vi "Handle Mouse Down.vi"(4 "PlatMods":T2, 6 "Mods":cluster{"Double Click":bool, "Menu Key":bool}, 8 "error in (no error)":errorcluster, 9 "Button":u16, 10 "Coords":T3, 11 "Process Builder View in":refnum<class "Process Builder View.lvclass">) -> (0 "error out":errorcluster, 2 "Mouse Down Filtered Event Data":T1, 3 "Process Builder View out":refnum<class "Process Builder View.lvclass">)   [LabVIEW 2019, in "Process Builder View.lvclass"]
uses:
  <vilib>/gpm_packages/@cs/Car-wash/Source/Process Builder View/Process Builder View.lvclass
  C:/Program Files/National Instruments/LabVIEW 2019/vi.lib/gpm_packages/@cs/Test-executive-builder/Source/Test Executive Builder View/Test Executive Builder View/Test Executive Builder View.lvclass
  <vilib>/Utility/miscctls.llb/LVPoint32TypeDef.ctl
  <vilib>/gpm_packages/@cs/Test-executive-builder/Source/Application Dependencies/Mouse Down Filtered Event Data.ctl
  <vilib>/gpm_packages/@cs/Test-executive-builder/Source/Test Executive Builder View/Test Executive Builder View/Test Executive Builder View.lvclass/Test Executive Builder View.ctl
  <vilib>/gpm_packages/@cs/Test-executive-builder/Source/Test Executive Builder View/Test Executive Builder View/Test Executive Builder View.lvclass
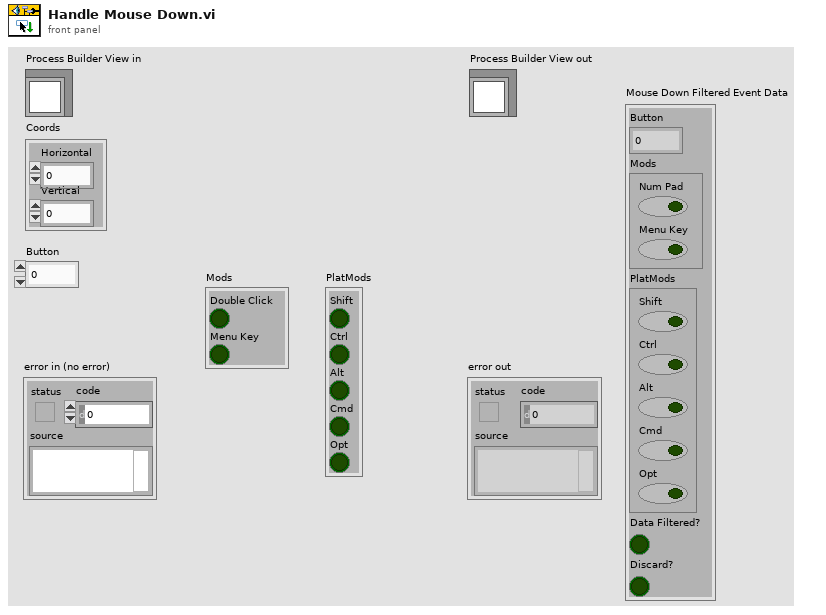
[diagram p1: front panel]
types:
  T1 = typedef "Mouse Down Filtered Event Data.ctl" = cluster{"Button":u16, "Mods":cluster{"Num Pad":bool, "Menu Key":bool}, "PlatMods":cluster{"Shift":bool, "Ctrl":bool, "Alt":bool, "Cmd":bool, "Opt":bool}, "Data Filtered?":bool, "Discard?":bool}
  T2 = cluster{"Shift":bool, "Ctrl":bool, "Alt":bool, "Cmd":bool, "Opt":bool}
  T3 = typedef "LVPoint32TypeDef.ctl" = cluster{"Horizontal":i32, "Vertical":i32}
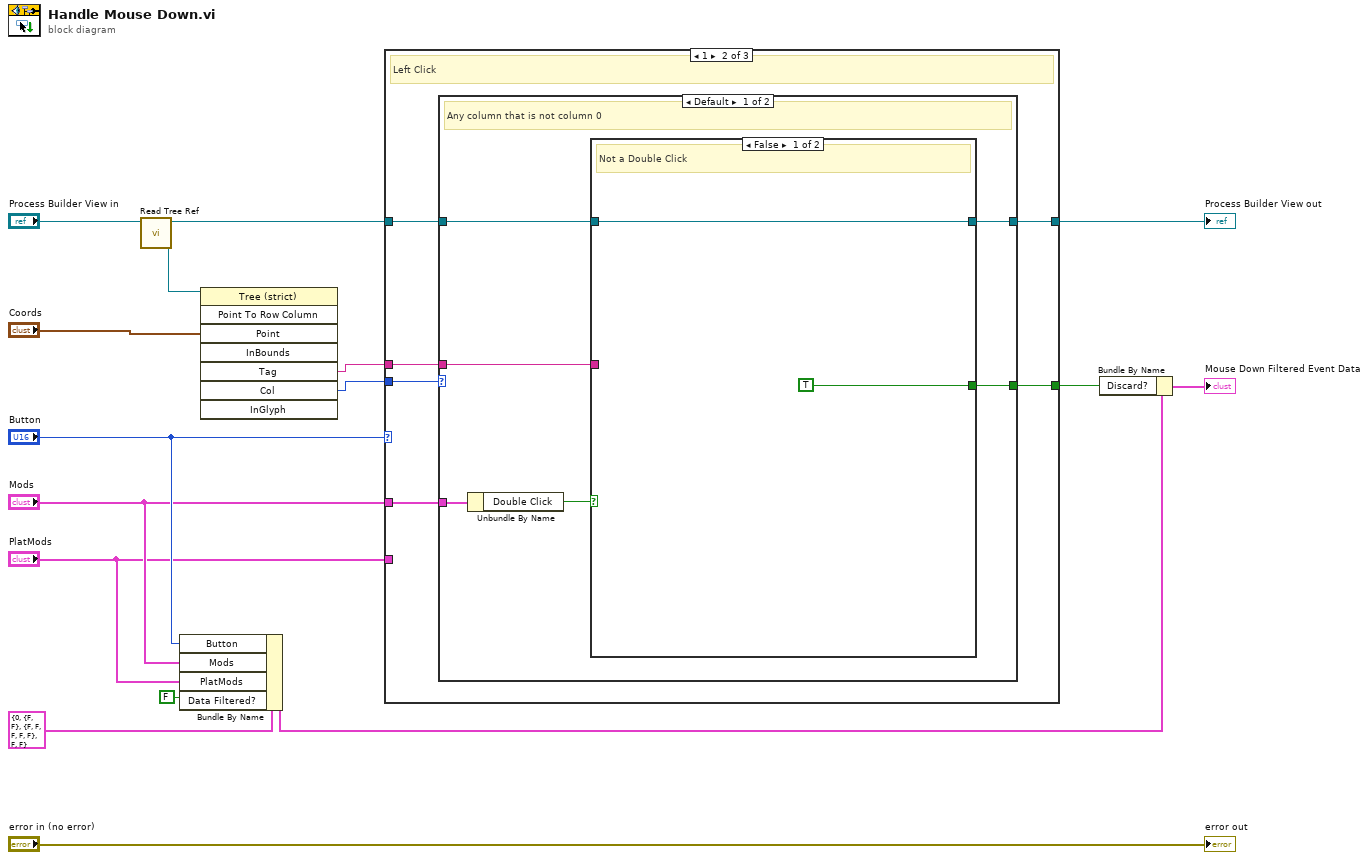
[diagram p0: block diagram]
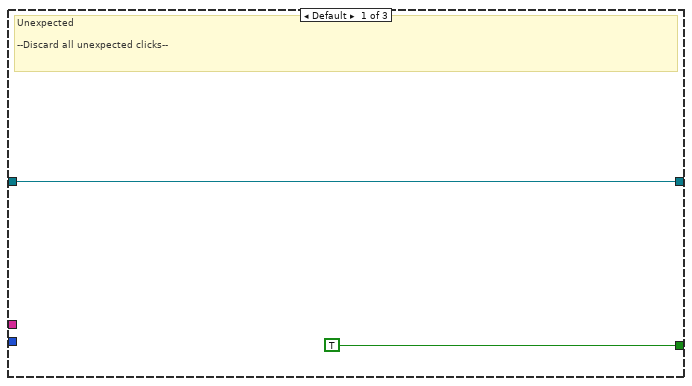
[diagram p2: hidden frame]
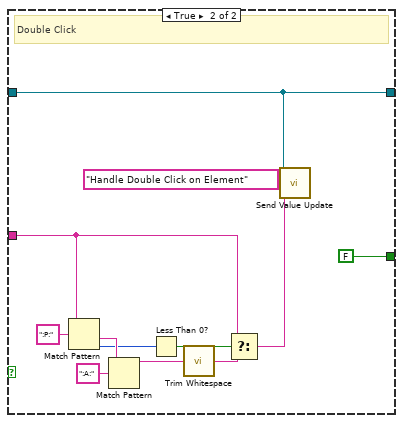
[diagram p3: hidden frame]
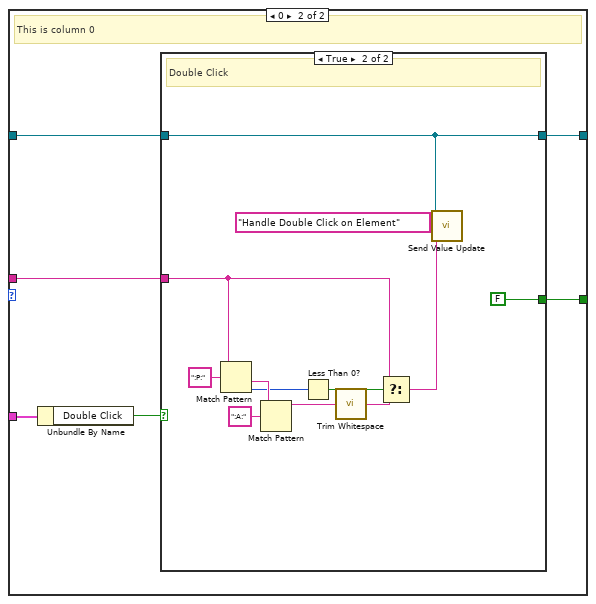
[diagram p4: hidden frame]
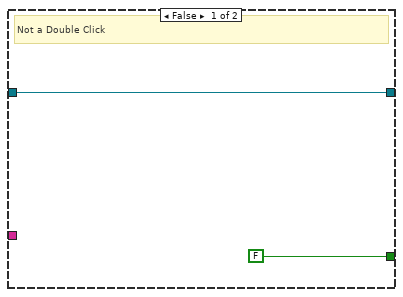
[diagram p5: hidden frame]
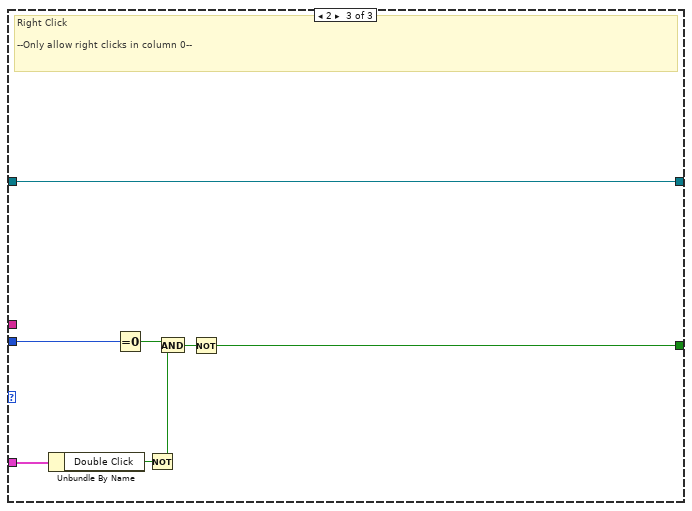
[diagram p6: hidden frame]
diagram:
  n1 = call <vilib>:"Read Tree Ref.vi"("Test Executive Builder View in"="Process Builder View in") -> ("Tree Ref"=w16:refnum<vi>, "Test Executive Builder View out"=w9:refnum<class "Process Builder View.lvclass">)  [unwired: 9 in]
  n2 = Bundle By Name(cluster=T1 {"Button"=0, "Mods"={"Num Pad"=FALSE, "Menu Key"=FALSE}, "PlatMods"={"Shift"=FALSE, "Ctrl"=FALSE, "Alt"=FALSE, "Cmd"=FALSE, "Opt"=FALSE}, "Data Filtered?"=FALSE, "Discard?"=FALSE} ("Mouse Down Filtered Event Data"), "Button"="Button", "Mods"="Mods", "PlatMods"="PlatMods", "Data Filtered?"=FALSE) -> (w12:T1)
  n3 = invoke class="Tree (strict)" method="Point To Row Column"(reference=w16, "Point"="Coords") -> ("Tag"=w14:string, "Col"=w15:i32)  [unwired: 6 in, 6 out]
  n4 = case shown="1" "Button" {
    tunnel: w15 -> [_ w24 w72]
    tunnel: w14 -> [_ w19 _]
    tunnel: "Mods" -> [_ w23 w70]
    tunnel: "PlatMods" -> [_ _ _]
    tunnel: [TRUE w22 w66] -> w10
    tunnel: w9 -> [w17 w21 w65]
    tunnel: [w17 w20 w65] -> w7
    frame Default {
      # "Unexpected\n\n--Discard all unexpected clicks--"
    }
    frame 1 {
      # "Left Click"
      n5 = case shown="Default" w24 {
        tunnel: w23 -> [w30 w50]
        tunnel: [w28 w48] -> w22
        tunnel: w21 -> [w26 w46]
        tunnel: [w27 w47] -> w20
        tunnel: w19 -> [w25 w45]
        frame Default {
          # "Any column that is not column 0"
          n6 = Unbundle By Name(w30) -> ("Double Click"=w29:bool)
          n7 = case shown="False" w29 {
            tunnel: [TRUE FALSE] -> w28
            tunnel: [w31 w35] -> w27
            tunnel: w26 -> [w31 w35]
            tunnel: w25 -> [_ w36]
            frame False {
              # "Not a Double Click"
            }
            frame True {
              # "Double Click"
              n8 = Match Pattern(string=w36, regular expression=":P:") -> (after substring=w42:string, offset past match=w41:i32)  [unwired: 1 in, 2 out]
              n9 = Match Pattern(string=w42, regular expression=":A:") -> (before substring=w40:string)  [unwired: 1 in, 3 out]
              n10 = Less Than 0?(x=w41) -> (x < 0?=w38:bool)
              n11 = call <vilib>:"Trim Whitespace.vi"("string"=w40) -> ("trimmed string"=w37:string)  [unwired: 1 in]
              n12 = Select(t=w36, s=w38, f=w37) -> (s? t:f=w34:string)
              n13 = call-dynamic "Send Value Update.vi"("Value"=w34, "Datum Name"="Handle Double Click on Element", "IViewable in"=w35) -> ()  [unwired: 8 in, 1 out]
            }
          }
        }
        frame 0 {
          # "This is column 0"
          n14 = Unbundle By Name(w50) -> ("Double Click"=w49:bool)
          n15 = case shown="True" w49 {
            tunnel: [FALSE FALSE] -> w48
            tunnel: [w51 w55] -> w47
            tunnel: w46 -> [w51 w55]
            tunnel: w45 -> [_ w56]
            frame False {
              # "Not a Double Click"
            }
            frame True {
              # "Double Click"
              n16 = Match Pattern(string=w56, regular expression=":P:") -> (after substring=w62:string, offset past match=w61:i32)  [unwired: 1 in, 2 out]
              n17 = Match Pattern(string=w62, regular expression=":A:") -> (before substring=w60:string)  [unwired: 1 in, 3 out]
              n18 = Less Than 0?(x=w61) -> (x < 0?=w58:bool)
              n19 = call <vilib>:"Trim Whitespace.vi"("string"=w60) -> ("trimmed string"=w57:string)  [unwired: 1 in]
              n20 = Select(t=w56, s=w58, f=w57) -> (s? t:f=w54:string)
              n21 = call-dynamic "Send Value Update.vi"("Value"=w54, "Datum Name"="Handle Double Click on Element", "IViewable in"=w55) -> ()  [unwired: 8 in, 1 out]
            }
          }
        }
      }
    }
    frame 2 {
      # "Right Click\n\n--Only allow right clicks in column 0--"
      n22 = Unbundle By Name(w70) -> ("Double Click"=w69:bool)
      n23 = Equal To 0?(x=w72) -> (x = 0?=w71:bool)
      n24 = Not(x=w69) -> (.not. x?=w68:bool)
      n25 = And(x=w71, y=w68) -> (x .and. y?=w67:bool)
      n26 = Not(x=w67) -> (.not. x?=w66:bool)
    }
  }
  "Process Builder View out" <- w7
  n27 = Bundle By Name(cluster=w12, "Discard?"=w10) -> (→"Mouse Down Filtered Event Data":T1)
  "error out" <- "error in (no error)"
